vi "Operation (SubVI).vi"(8 "error in (no error)":errorcluster, 9 "On/Off":bool=TRUE, 10 "Operation":T1(ring), 11 "DAQmx Device Name":tag) -> (0 "error out":errorcluster)   [LabVIEW 2017]
uses:
  <vilib>/DAQmx/write.llb/DAQmx Write (Digital Bool 1Line 1Point).vi
  <vilib>/DAQmx/create/channels.llb/DAQmx Create Channel (DO-Digital Output).vi
panel:
  in  "lines":tag
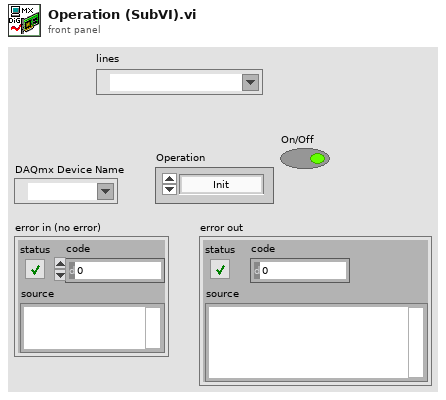
[diagram p1: front panel]
types:
  T1 = enum16{"Init", "0 ohm", "6 ohm", "13.2 ohm", "15 ohm", "25.9 ohm", "33 ohm", "Down", "Up", "Venable", "Firmware", "PowerSuply"}
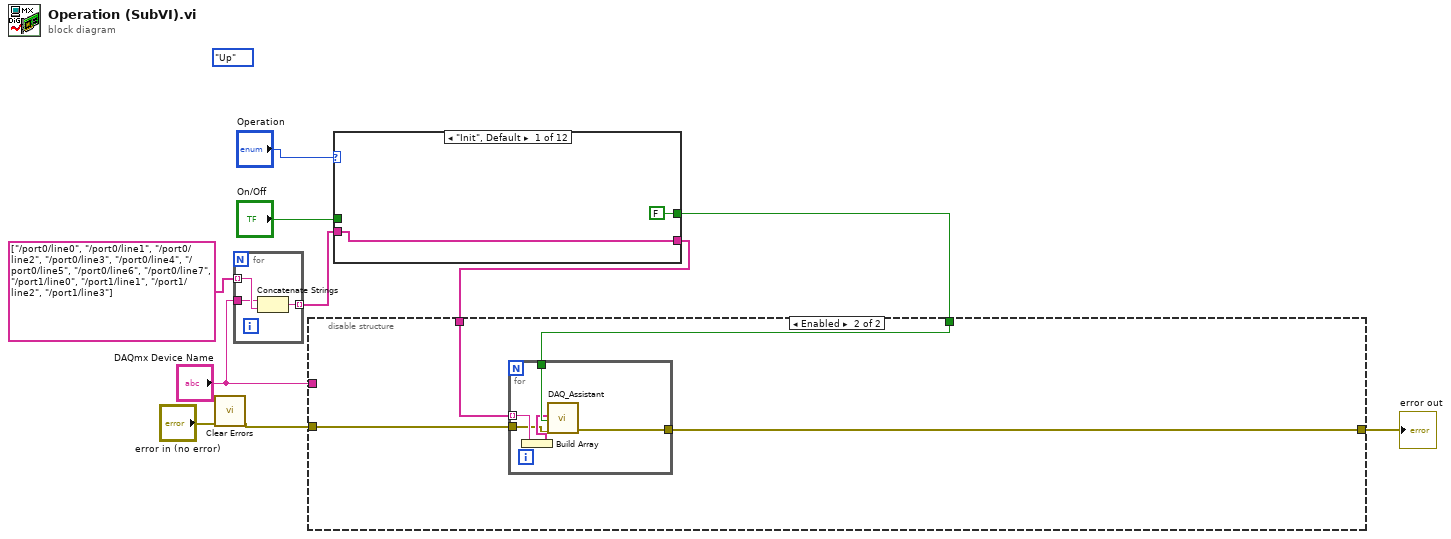
[diagram p0: block diagram]
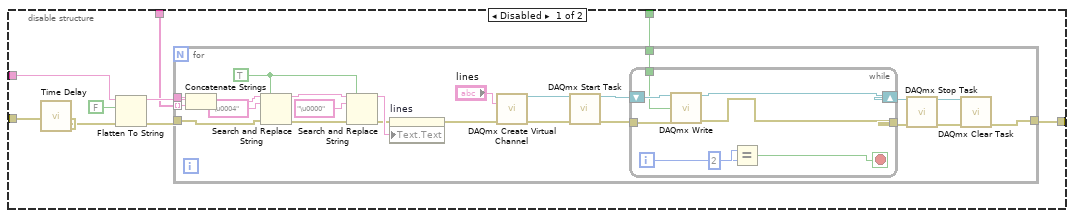
[diagram p2: hidden frame]
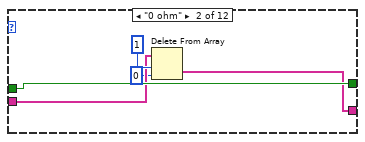
[diagram p3: hidden frame]
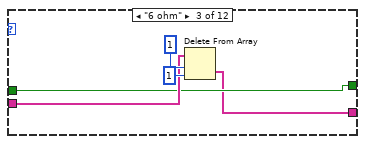
[diagram p4: hidden frame]
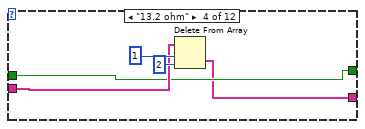
[diagram p5: hidden frame]
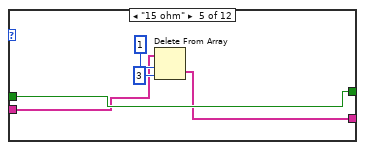
[diagram p6: hidden frame]
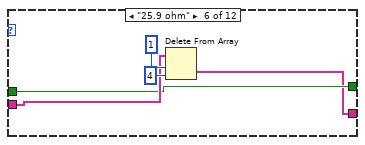
[diagram p7: hidden frame]
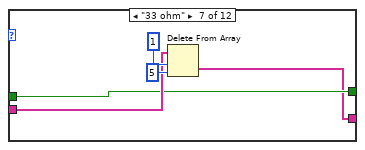
[diagram p8: hidden frame]
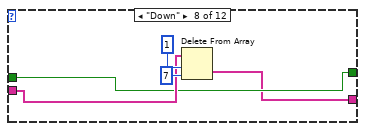
[diagram p9: hidden frame]
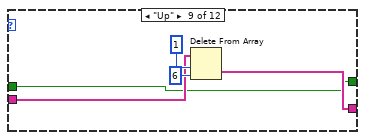
[diagram p10: hidden frame]
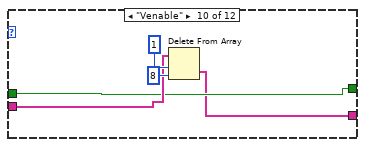
[diagram p11: hidden frame]
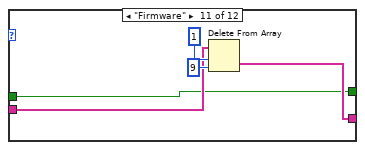
[diagram p12: hidden frame]
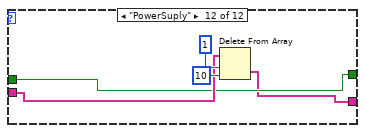
[diagram p13: hidden frame]
diagram:
  (unwired) T1."Up" ("Operation 2")
  n1 = call <vilib>:"Clear Errors.vi"("error in (no error)"="error in (no error)") -> ("error out"=w1:errorcluster)  [unwired: 5 in, 1 out]
  n2 = for {
    tunnel: string[] ["/port0/line0", "/port0/line1", "/port0/line2", "/port0/line3", "/port0/line4", "/port0/line5", "/port0/line6", "/port0/line7", "/port1/line0", "/port1/line1", "/port1/line2", "/port1/line3"] -> [w13] mode=indexing
    tunnel: "DAQmx Device Name" -> [w12]
    tunnel: [w11] -> w2 mode=indexing
    n3 = Concatenate Strings(w12, w13) -> (w11:string)
  }
  n4 = case shown="\"Init\", Default" "Operation" {
    tunnel: "On/Off" -> [_ w20 w22 w27 w33 w37 w42 w47 w51 w57 w61 w67]
    tunnel: [FALSE ("On/Off") w20 w22 w27 w33 w37 w42 w47 w51 w57 w61 w67] -> w6
    tunnel: [w14 w16 w21 w26 w31 w36 w41 w46 w52 w56 w62 w66] -> w5
    tunnel: w2 -> [w14 w18 w23 w28 w32 w38 w43 w48 w53 w58 w63 w68]
    frame "Init", Default {
    }
    frame "0 ohm" {
      n5 = Delete From Array(array=w18, length=1, index=0) -> (deleted portion=w16:string[])  [unwired: 1 out]
    }
    frame "6 ohm" {
      n6 = Delete From Array(array=w23, length=1, index=1) -> (deleted portion=w21:string[])  [unwired: 1 out]
    }
    frame "13.2 ohm" {
      n7 = Delete From Array(array=w28, length=1, index=2) -> (deleted portion=w26:string[])  [unwired: 1 out]
    }
    frame "15 ohm" {
      n8 = Delete From Array(array=w32, length=1, index=3) -> (deleted portion=w31:string[])  [unwired: 1 out]
    }
    frame "25.9 ohm" {
      n9 = Delete From Array(array=w38, length=1, index=4) -> (deleted portion=w36:string[])  [unwired: 1 out]
    }
    frame "33 ohm" {
      n10 = Delete From Array(array=w43, length=1, index=5) -> (deleted portion=w41:string[])  [unwired: 1 out]
    }
    frame "Down" {
      n11 = Delete From Array(array=w48, length=1, index=7) -> (deleted portion=w46:string[])  [unwired: 1 out]
    }
    frame "Up" {
      n12 = Delete From Array(array=w53, length=1, index=6) -> (deleted portion=w52:string[])  [unwired: 1 out]
    }
    frame "Venable" {
      n13 = Delete From Array(array=w58, length=1, index=8) -> (deleted portion=w56:string[])  [unwired: 1 out]
    }
    frame "Firmware" {
      n14 = Delete From Array(array=w63, length=1, index=9) -> (deleted portion=w62:string[])  [unwired: 1 out]
    }
    frame "PowerSuply" {
      n15 = Delete From Array(array=w68, length=1, index=10) -> (deleted portion=w66:string[])  [unwired: 1 out]
    }
  }
  n16 = disable-structure shown="Enabled" {
    disable-tunnel: w1 -> [w77 w111]
    disable-tunnel: [w75 w112] -> w7
    disable-tunnel: w6 -> [w74 w113]
    disable-tunnel: w5 -> [w73 w114]
    disable-tunnel: "DAQmx Device Name" -> [w71 _]
    frame Disabled {
      n17 = call "Time Delay"("error in (no error)"=w77) -> ("error out"=w72:errorcluster)  [unwired: 10 in]
      n18 = Flatten To String(anything=w71, prepend array or string size? (T)=FALSE, error in (no error)=w72) -> (data string=w79:string, error out=w76:errorcluster)  [unwired: 1 in, 1 out]
      n19 = for {
        tunnel: w79 -> [w102]
        tunnel: w74 -> [w86]
        tunnel: w76 -> [w91]
        tunnel: [w81] -> w75
        tunnel: w73 -> [w85] mode=indexing
        w92 = TRUE ("replace all? (F)")
        n20 = Concatenate Strings(w102, w85) -> (w97:string)
        n21 = Search and Replace String(replace all?=w92, input string=w97, search string="\u0004", error in=w91) -> (result string=w94:string, error out=w90:errorcluster)  [unwired: 4 in, 2 out]
        n22 = Search and Replace String(replace all?=w92, input string=w94, search string="\u0000", error in=w90) -> (result string=w93:string, error out=w89:errorcluster)  [unwired: 4 in, 2 out]
        n23 = property on="lines" class="DAQmxName"(error in=w89, "Text.Text"=w93) -> (error out=w98:errorcluster)  [unwired: 1 in, 1 out]
        n24 = call-poly <vilib>:"DAQmx Create Virtual Channel.vi"("lines"="lines", "error in"=w98) -> ("task out"=w101:refnum<k21>, "error out"=w88:errorcluster)  [unwired: 12 in]
        n25 = call <vilib>:"DAQmx Start Task.vi"("task/channels in"=w101, "error in"=w88) -> ("task out"=w100:refnum<k21>, "error out"=w87:errorcluster)  [unwired: 12 in]
        n26 = while {
          tunnel: w86 -> [w103]
          shift-right: [w108] -> w84
          shift-left: w100 -> [w110]
          tunnel: w87 -> [w109]
          tunnel: [w107] -> w83
          i -> [w106]
          stop <- w104 stop-if-true
          n27 = call-poly <vilib>:"DAQmx Write.vi"("task/channels in"=w110, "data"=w103, "error in"=w109) -> ("task out"=w108:refnum<k21>, "error out"=w107:errorcluster)  [unwired: 10 in, 1 out]
          n28 = Equal?(x=w106, y=2) -> (x = y?=w104:bool)
        }
        n29 = call <vilib>:"DAQmx Stop Task.vi"("task/channels in"=w84, "error in"=w83) -> ("task out"=w80:refnum<k21>, "error out"=w82:errorcluster)  [unwired: 12 in]
        n30 = call <vilib>:"DAQmx Clear Task.vi"("task in"=w80, "error in"=w82) -> ("error out"=w81:errorcluster)  [unwired: 13 in]
      }
    }
    frame Enabled {
      n31 = for {
        tunnel: w114 -> [w117] mode=indexing
        tunnel: w113 -> [w119]
        tunnel: [w118] -> w112
        tunnel: w111 -> [w115]
        n32 = Build Array(w117) -> (w116:string[])
        n33 = call "DAQ_Assistant.vi"("Lines"=w116, "data 2"=w119, "error in"=w115) -> ("error out"=w118:errorcluster)  [unwired: 15 in, 1 out]
      }
    }
  }
  "error out" <- w7
